vi "Chroma.vi"(11 "resource name":refnum<k15>) -> (1 "VA":dbl[](array[numeric]), 2 "Current":dbl[](array[numeric]), 3 "Voltage":dbl[](array[numeric]))   [LabVIEW 2015]
panel:
  out "VAR":dbl caption="Read Value"
  out "I_THD":dbl caption="Read Value"
  out "I_PP+":dbl caption="Read Value"
  out "I_PP-":dbl caption="Read Value"
  out "V_THD":dbl caption="Read Value"
  out "V_PP+":dbl caption="Read Value"
  out "V_PP-":dbl caption="Read Value"
  out "Frequency":dbl caption="Read Value"
  out "Power Factor":dbl[](array[numeric])
  out "Watts":dbl[](array[numeric])
  in  "stop":bool
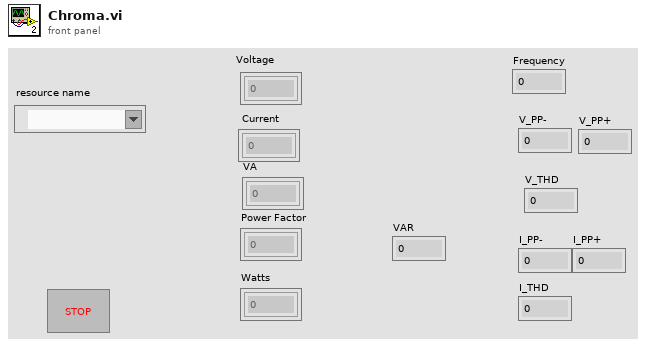
[diagram p1: front panel]
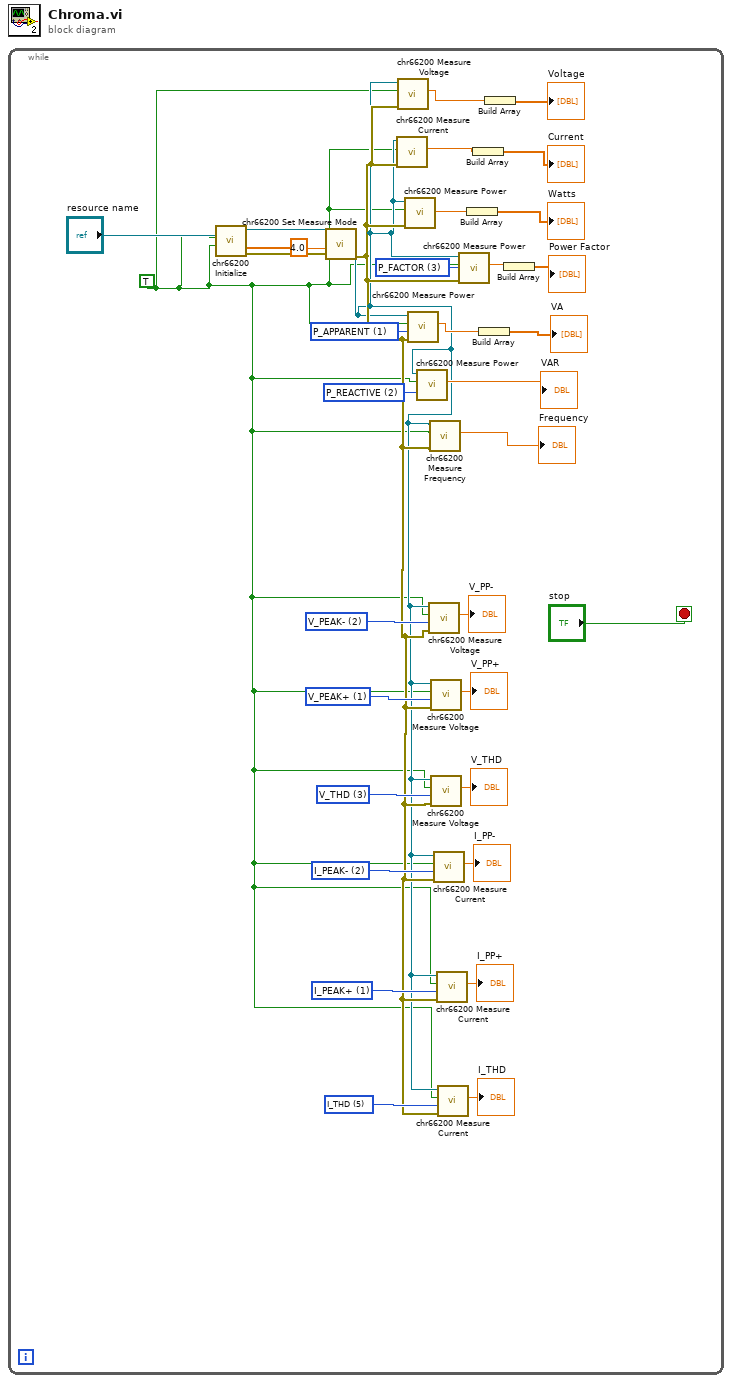
[diagram p0: block diagram]
diagram:
  n1 = while {
    stop <- "stop" stop-if-true
    w8 = 5 items=["I_THD"=5, "I_CRESTFACTOR"=4, "I_INRUSH"=3, "I_PEAK-"=2, "I_PEAK+"=1, "I_RMS"=0] ("Type (I_RMS)")
    w9 = 1 items=["I_THD"=5, "I_CRESTFACTOR"=4, "I_INRUSH"=3, "I_PEAK-"=2, "I_PEAK+"=1, "I_RMS"=0] ("Type (I_RMS)")
    w10 = 2 items=["I_THD"=5, "I_CRESTFACTOR"=4, "I_INRUSH"=3, "I_PEAK-"=2, "I_PEAK+"=1, "I_RMS"=0] ("Type (I_RMS)")
    w14 = 3 items=["V_THD"=3, "V_PEAK-"=2, "V_PEAK+"=1, "V_RMS"=0] ("Type (V_RMS)")
    w15 = 1 items=["V_THD"=3, "V_PEAK-"=2, "V_PEAK+"=1, "V_RMS"=0] ("Type (V_RMS)")
    w17 = 2 items=["P_ENERGY"=4, "P_FACTOR"=3, "P_REACTIVE"=2, "P_APPARENT"=1, "P_REAL"=0] ("Type (P_REAL)")
    w16 = 2 items=["V_THD"=3, "V_PEAK-"=2, "V_PEAK+"=1, "V_RMS"=0] ("Type (V_RMS)")
    w22 = 1 items=["P_ENERGY"=4, "P_FACTOR"=3, "P_REACTIVE"=2, "P_APPARENT"=1, "P_REAL"=0] ("Type (P_REAL)")
    w23 = 3 items=["P_ENERGY"=4, "P_FACTOR"=3, "P_REACTIVE"=2, "P_APPARENT"=1, "P_REAL"=0] ("Type (P_REAL)")
    w1 = TRUE
    n2 = call <instrlib>:"chr66200 Initialize.vi"("Reset Device (Yes)"=w1, "ID Query (Yes)"=w1, "resource name"="resource name") -> ("error out"=w31:errorcluster, "instrument handle out"=w34:refnum<k15>)  [unwired: 7 in]
    n3 = call <instrlib>:"chr66200 Set Measure Mode.vi"("error in (no error)"=w31, "Window Time (4)"=4.0, "Measure Mode (Window)"=w1, "instrument handle"=w34) -> ("error out"=w7:errorcluster, "instrument handle out"=w2:refnum<k15>)  [unwired: 6 in]
    n4 = call <instrlib>:"chr66200 Measure Current.vi"("error in (no error)"=w7, "Measure Fetch (Fetch)"=w1, "instrument handle"=w2) -> ("Read Value"=w29:dbl)  [unwired: 6 in, 2 out]
    n5 = call <instrlib>:"chr66200 Measure Voltage.vi"("error in (no error)"=w7, "Measure Fetch (Fetch)"=w1, "instrument handle"=w2) -> ("Read Value"=w19:dbl)  [unwired: 6 in, 2 out]
    n6 = call <instrlib>:"chr66200 Measure Power.vi"("error in (no error)"=w7, "Measure Fetch (Fetch)"=w1, "instrument handle"=w2) -> ("Read Value"=w27:dbl)  [unwired: 6 in, 2 out]
    n7 = call <instrlib>:"chr66200 Measure Power.vi"("error in (no error)"=w7, "Type (P_REAL)"=w22, "Measure Fetch (Fetch)"=w1, "instrument handle"=w2) -> ("Read Value"=w20:dbl)  [unwired: 5 in, 2 out]
    n8 = call <instrlib>:"chr66200 Measure Power.vi"("Type (P_REAL)"=w17, "Measure Fetch (Fetch)"=w1, "instrument handle"=w2) -> ("Read Value"=→"VAR":dbl)  [unwired: 6 in, 2 out]
    n9 = call <instrlib>:"chr66200 Measure Voltage.vi"("error in (no error)"=w7, "Type (V_RMS)"=w16, "Measure Fetch (Fetch)"=w1, "instrument handle"=w2) -> ("Read Value"=→"V_PP-":dbl)  [unwired: 5 in, 2 out]
    n10 = call <instrlib>:"chr66200 Measure Frequency.vi"("error in (no error)"=w7, "Measure Fetch (Fetch)"=w1, "instrument handle"=w2) -> ("Read Value"=→"Frequency":dbl)  [unwired: 6 in, 2 out]
    n11 = call <instrlib>:"chr66200 Measure Voltage.vi"("error in (no error)"=w7, "Type (V_RMS)"=w15, "Measure Fetch (Fetch)"=w1, "instrument handle"=w2) -> ("Read Value"=→"V_PP+":dbl)  [unwired: 5 in, 2 out]
    n12 = call <instrlib>:"chr66200 Measure Voltage.vi"("error in (no error)"=w7, "Type (V_RMS)"=w14, "Measure Fetch (Fetch)"=w1, "instrument handle"=w2) -> ("Read Value"=→"V_THD":dbl)  [unwired: 5 in, 2 out]
    n13 = call <instrlib>:"chr66200 Measure Current.vi"("error in (no error)"=w7, "Type (I_RMS)"=w10, "Measure Fetch (Fetch)"=w1, "instrument handle"=w2) -> ("Read Value"=→"I_PP-":dbl)  [unwired: 5 in, 2 out]
    n14 = call <instrlib>:"chr66200 Measure Current.vi"("error in (no error)"=w7, "Type (I_RMS)"=w9, "Measure Fetch (Fetch)"=w1, "instrument handle"=w2) -> ("Read Value"=→"I_PP+":dbl)  [unwired: 5 in, 2 out]
    n15 = call <instrlib>:"chr66200 Measure Current.vi"("error in (no error)"=w7, "Type (I_RMS)"=w8, "Measure Fetch (Fetch)"=w1, "instrument handle"=w2) -> ("Read Value"=→"I_THD":dbl)  [unwired: 5 in, 2 out]
    n16 = call <instrlib>:"chr66200 Measure Power.vi"("error in (no error)"=w7, "Type (P_REAL)"=w23, "Measure Fetch (Fetch)"=w1, "instrument handle"=w2) -> ("Read Value"=w25:dbl)  [unwired: 5 in, 2 out]
    n17 = Build Array(w27) -> (→"Watts":dbl[])
    n18 = Build Array(w29) -> (→"Current":dbl[])
    n19 = Build Array(w20) -> (→"VA":dbl[])
    n20 = Build Array(w19) -> (→"Voltage":dbl[])
    n21 = Build Array(w25) -> (→"Power Factor":dbl[])
  }
